vi "Wave1D_Cal U_Apply BC.vi"(6 "time step":i32, 8 "length":i32, 9 "End X Value":dbl[](array[numeric]), 10 "Start X Value":dbl[](array[numeric]), 11 "U In":dbl[](array[numeric])) -> (3 "U Out":dbl[](array[numeric]))   [LabVIEW 2020, in "NI_PDE.lvlib"]
uses:
  <vilib>/gmath/NI_PDE.lvlib
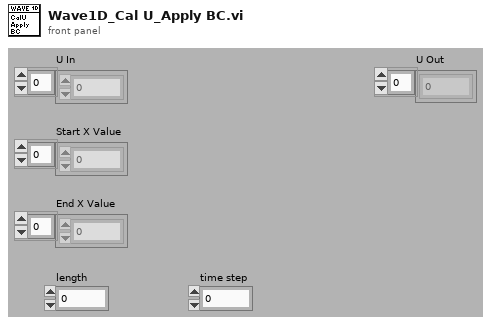
[diagram p1: front panel]
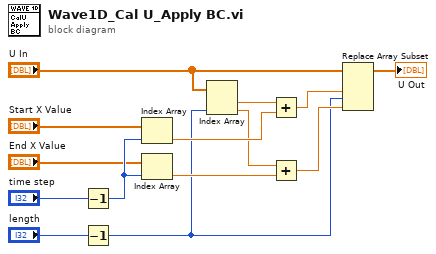
[diagram p0: block diagram]
diagram:
  n1 = Decrement(x="time step") -> (x-1=w6:i32)
  n2 = Decrement(x="length") -> (x-1=w8:i32)
  n3 = Index Array(array="Start X Value", index=w6) -> (element=w13:dbl)
  n4 = Index Array(array="End X Value", index=w6) -> (element=w11:dbl)
  n5 = Index Array(array="U In", index #2=w8) -> (element #1=w14:dbl, element #2=w12:dbl)  [unwired: 1 in]
  n6 = Add(x=w14, y=w13) -> (x+y=w10:dbl)
  n7 = Add(x=w12, y=w11) -> (x+y=w9:dbl)
  n8 = Replace Array Subset(array="U In", new element #1=w10, new element #2=w9, index #2=w8) -> (→"U Out":dbl[])  [unwired: 1 in]
